vi "Log Event.vi"(8 "error in (no error)":errorcluster, 10 "Event Text":string, 11 "AFTest in":refnum<class "AFTest.lvclass">) -> (0 "error out":errorcluster)   [LabVIEW 2014, in "AFTest.lvlib" / "AFTest.lvclass"]
doc: "Add text to the ongoing event log."
uses:
  AFTest.lvclass
  AFTest.lvclass/AFTest.ctl
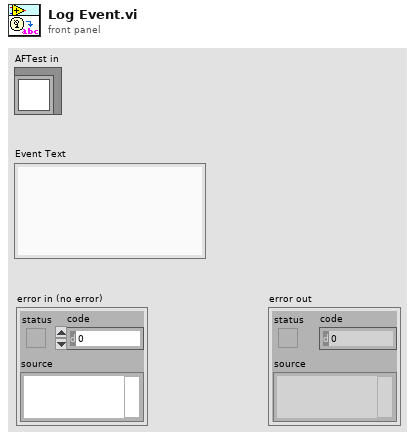
[diagram p1: front panel]
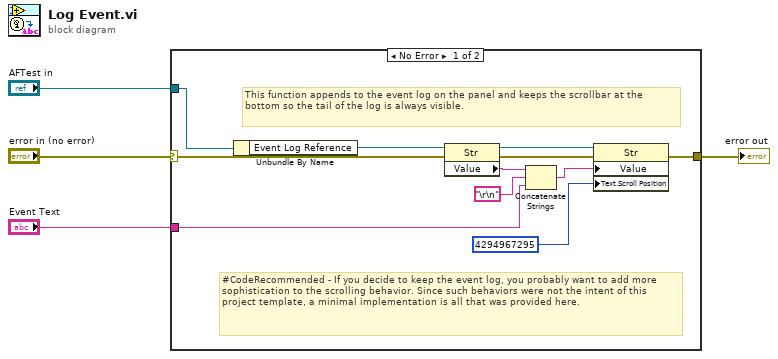
[diagram p0: block diagram]
diagram:
  n1 = case shown="No Error" "error in (no error)" {
    selector: "error in (no error)" -> [w7 w16]
    tunnel: [w8 w16] -> w3
    tunnel: "AFTest in" -> [w15 _]
    tunnel: "Event Text" -> [w12 _]
    frame No Error {
      # "#CodeRecommended - If you decide to keep the event log, you probably want to add more sophistication to the scrolling behavior. Since such behaviors were not the intent of this project template, a minimal implementation is all that was provided here."
      # "This function appends to the event log on the panel and keeps the scrollbar at the bottom so the tail of the log is always visible."
      n2 = Unbundle By Name(w15) -> ("Event Log Reference"=w14:refnum<vi>)
      n3 = property class="Str"(reference=w14, error in=w7) -> (reference out=w10:refnum<vi>, error out=w9:errorcluster, "Value"=w13:string)
      n4 = Concatenate Strings(w13, "\r\n", w12) -> (w6:string)
      n5 = property class="Str"(reference=w10, error in=w9, "Value"=w6, "Text.Scroll Position"=u32 4294967295) -> (error out=w8:errorcluster)  [unwired: 1 out]
    }
    frame Error {
    }
  }
  "error out" <- w3
